vi "Configure Frequency (Center Span).vi"(8 "error in (no error)":errorcluster, 9 "Span (2 GHz)":dbl=2000000000.0, 10 "Center Frequency (2 GHz)":dbl=2000000000.0, 11 "VISA resource name":refnum<visa-resource-name>) -> (0 "error out":errorcluster, 3 "VISA resource name out":refnum<visa-resource-name>)   [LabVIEW 2014]
uses:
  Agilent ESA PSA Series.lvlib
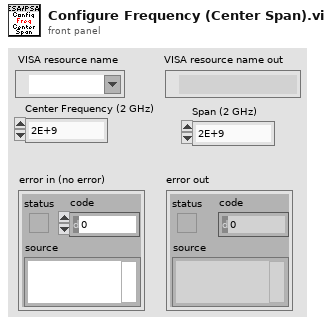
[diagram p1: front panel]
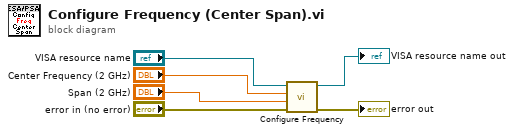
[diagram p0: block diagram]
diagram:
  n1 = call-poly "Configure Frequency.vi"("error in (no error)"="error in (no error)", "Span (2 GHz)"="Span (2 GHz)", "Center Frequency (2 GHz)"="Center Frequency (2 GHz)", "VISA resource name"="VISA resource name") -> ("error out"=→"error out":errorcluster, "VISA resource name out"=→"VISA resource name out":refnum<visa-resource-name>)  [unwired: 6 in]
